vi "PCO_GetErrorText.vi"(8 "error in (no error)":errorcluster, 11 "Errorcode":u32 format="%x") -> (0 "error out":errorcluster, 3 "Error Out":u32 format="%.0x", 5 "return type":u32 format="%x")   [LabVIEW 2011]
uses:
  SC2_Cam64.dll
panel:
  out "Text":string
  # "bytes?"
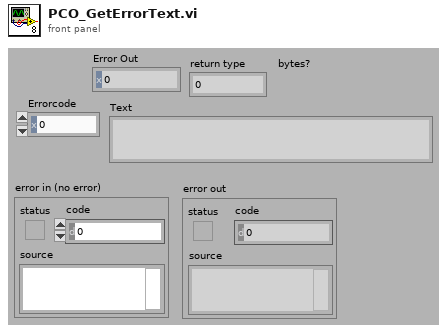
[diagram p1: front panel]
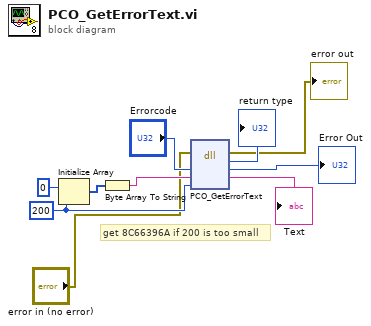
[diagram p0: block diagram]
diagram:
  w4 = u32 200
  # "get 8C66396A if 200 is too small"
  n1 = Initialize Array(u8 0 ("element"), w4) -> (w6:u8[])
  n2 = Byte Array To String(unsigned byte array=w6) -> (string=w5:string)
  n3 = dll-call lib="C:/Program Files/colibri/Drivers/PCO.Camera/SC2_Cam*.*" fn="PCO_GetErrorText"(error in="error in (no error)", "dwerr"="Errorcode", "Text"=w5, "TextBufferLength"=w4) -> (error out=→"error out":errorcluster, "return type"=→"return type":u32, "dwerr"=→"Error Out":u32, "Text"=→"Text":string)  [unwired: 3 in, 1 out]
